vi "ActivateReader.vi"(11 "PN 532 COM Port":refnum<visa-resource-name>) -> (0 "Error Out":errorcluster, 2 "Success?":bool, 3 "PN532 COM Port Out":refnum<visa-resource-name>)   [LabVIEW 2012, in "NFC Driver.lvlib"]
doc: "This VI wakes up and sets to Normal mode the PN532 at the COM Port specified by \"PN532 COM Port\" and then verifies that the target was succesfully activated by verifying the target's response."
uses:
  NFC Driver.lvlib
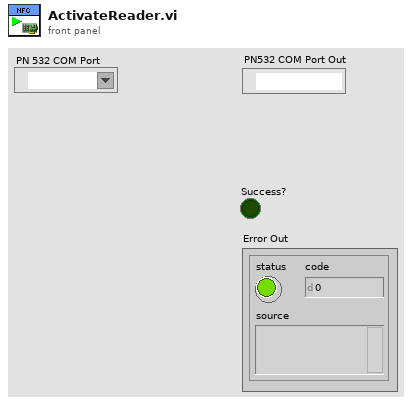
[diagram p1: front panel]
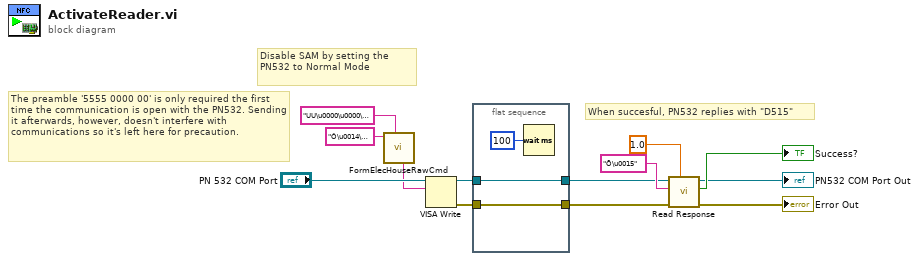
[diagram p0: block diagram]
diagram:
  # "The preamble '5555 0000 00' is only required the first time the communication is open with the PN532. Sending it afterwards, however, doesn't interfere with communications so it's left here for precaution."
  # "When succesful, PN532 replies with \"D515\""
  # "Disable SAM by setting the PN532 to Normal Mode"
  n1 = call "FormElecHouseRawCmd.vi"("Preamble"="UU\u0000\u0000\u0000", "Command"="Ô\u0014\u0001" ("NXP Command")) -> ("concatenated Cmd"=w11:string)  [unwired: 9 in]
  n2 = VISA Write(VISA resource name="PN 532 COM Port", write buffer=w11) -> (VISA resource name out=w9:refnum<visa-resource-name>, error out=w10:errorcluster)  [unwired: 1 in, 1 out]
  n3 = flat-sequence {
    tunnel: w10 -> [w14]
    tunnel: w9 -> [w15]
    tunnel: [w15] -> w5
    tunnel: [w14] -> w8
    frame #0 {
      n4 = Wait (ms)(milliseconds to wait=u32 100) -> ()  [unwired: 1 out]
    }
  }
  n5 = call "Read Response.vi"("Timeout (s)"=1.0, "error in (no error)"=w8, "regular expression"="Õ\u0015", "PN532 COM Port"=w5) -> ("error out"=→"Error Out":errorcluster, "Found?"=→"Success?":bool, "PN532 COM Port Out"=→"PN532 COM Port Out":refnum<visa-resource-name>)  [unwired: 4 in, 1 out]
